vi "EditSine.vi"() -> ()   [LabVIEW 2020, in "Curve Editor.lvlib"]
uses:
  Curve Editor.lvlib
  Key Value/Key Value.lvlib
panel:
  in  "偏移量":dbl format="%.2f"
  in  "相位[度]":dbl format="%.2f"
  in  "幅值":dbl format="%.2f"
  in  "频率":dbl format="%.2f"
  in  "时间[S]":dbl format="%.2f"
  in  "Tree引用句柄":refnum<vi>
  in  "索引":i32
  in  "取消按钮":bool
  in  "确定按钮":bool
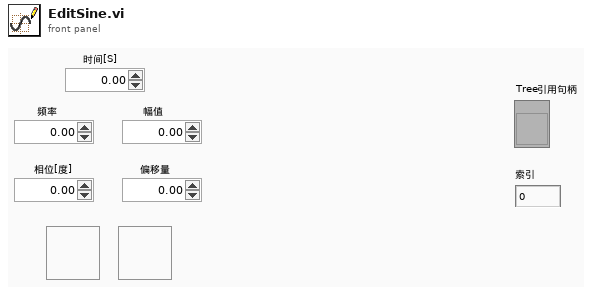
[diagram p1: front panel]
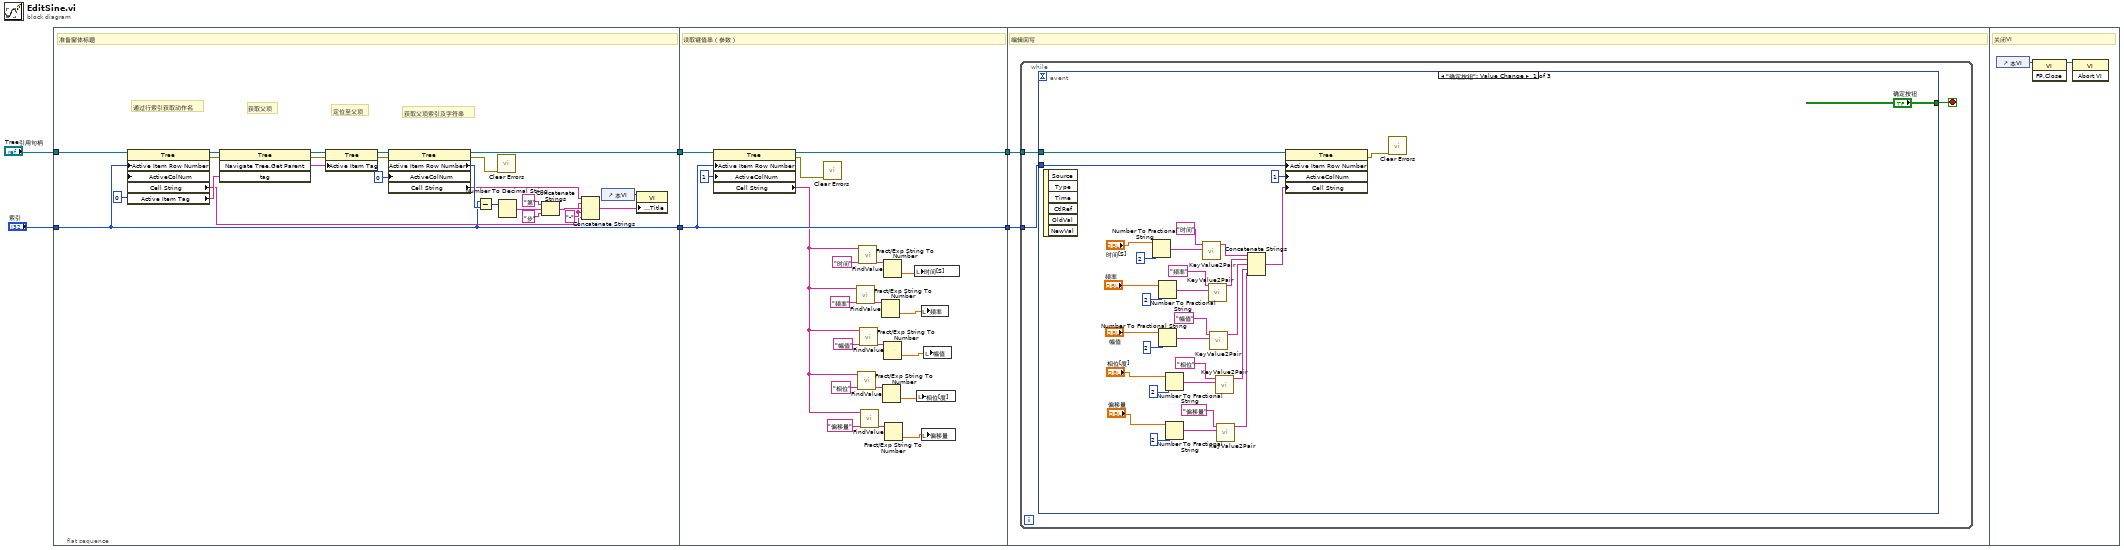
[diagram p0: block diagram]
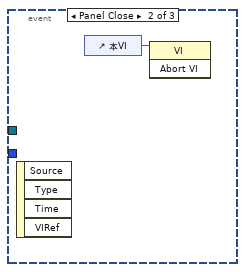
[diagram p2: hidden frame]
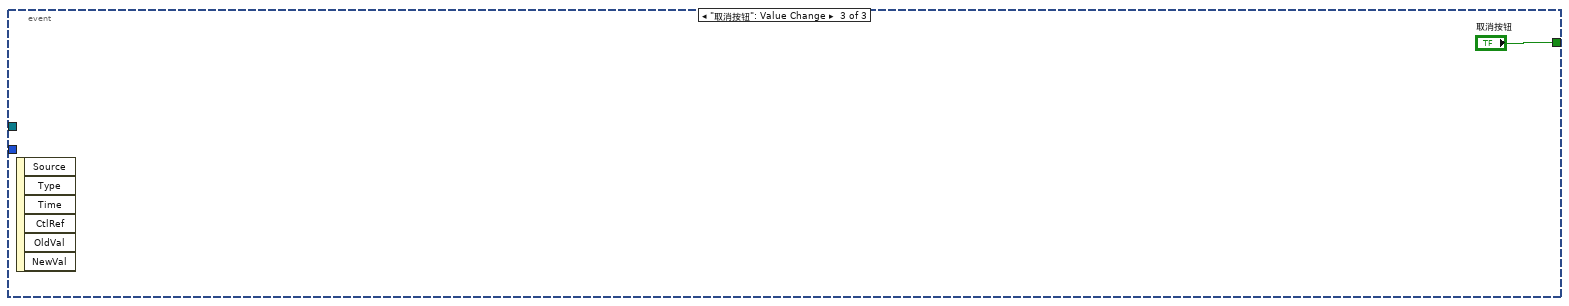
[diagram p3: hidden frame]
diagram:
  n1 = flat-sequence {
    tunnel: [w13] -> w6
    tunnel: [w12] -> w4
    tunnel: "Tree引用句柄" -> [w14]
    tunnel: "索引" -> [w13]
    tunnel: w6 -> [w50]
    tunnel: [w50] -> w5
    tunnel: w4 -> [w51]
    tunnel: [w49] -> w3
    tunnel: w5 -> [w54]
    tunnel: w3 -> [w53]
    frame #0 {
      w16 = "-" ("字符串")
      # "获取父项索引及字符串"
      # "定位至父项"
      # "获取父项"
      # "通过行索引获取动作名"
      # "准备窗体标题"
      n2 = property class="Tree"(reference=w14, "Active Item Row Number"=w13, "ActiveColNum"=0 ("活动单元格:活动列数")) -> (reference out=w11:refnum<vi>, error out=w10:errorcluster, "Cell String"=w15:string, "Active Item Tag"=w28:string)  [unwired: 1 in]
      n3 = invoke class="Tree" method="Navigate Tree.Get Parent"(reference=w11, error in=w10, "tag"=w28) -> (reference out=w23:refnum<vi>, error out=w9:errorcluster, "Navigate Tree:Get Parent"=w24:string)  [unwired: 1 in, 1 out]
      n4 = property class="Tree"(reference=w23, error in=w9, "Active Item Tag"=w24) -> (reference out=w22:refnum<vi>, error out=w8:errorcluster)
      n5 = property class="Tree"(reference=w22, error in=w8, "ActiveColNum"=0 ("活动单元格:活动列数")) -> (reference out=w12:refnum<vi>, error out=w7:errorcluster, "Active Item Row Number"=w26:i32, "Cell String"=w25:string)
      n6 = Subtract(x=w13, y=w26) -> (x-y=w21:i32)
      n7 = call <vilib>:"Clear Errors.vi"("error in (no error)"=w7) -> ()  [unwired: 5 in, 2 out]
      n8 = Number To Decimal String(number=w21) -> (decimal integer string=w19:string)  [unwired: 1 in]
      n9 = Concatenate Strings("第", w19, "步") -> (w17:string)
      n10 = Concatenate Strings(w25, w16, w17, w16, w15) -> (w29:string)
      n11 = control-ref of="本VI"() -> (w31:refnum<vi>)
      n12 = property class="VI"(reference=w31, "Front Panel.Title"=w29) -> ()  [unwired: 1 in, 2 out]
    }
    frame #1 {
      # "读取键值串（参数）"
      n13 = property class="Tree"(reference=w51, "Active Item Row Number"=w50, "ActiveColNum"=1 ("活动单元格:活动列数")) -> (reference out=w49:refnum<vi>, error out=w32:errorcluster, "Cell String"=w33:string)  [unwired: 1 in]
      n14 = call <vilib>:"Clear Errors.vi"("error in (no error)"=w32) -> ()  [unwired: 5 in, 2 out]
      n15 = call "FindValue.vi"("键"="频率", "键值串"=w33) -> ("值"=w44:string)  [unwired: 8 in, 1 out]
      n16 = call "FindValue.vi"("键"="相位", "键值串"=w33) -> ("值"=w38:string)  [unwired: 8 in, 1 out]
      n17 = call "FindValue.vi"("键"="时间", "键值串"=w33) -> ("值"=w47:string)  [unwired: 8 in, 1 out]
      n18 = call "FindValue.vi"("键"="幅值", "键值串"=w33) -> ("值"=w41:string)  [unwired: 8 in, 1 out]
      n19 = call "FindValue.vi"("键"="偏移量", "键值串"=w33) -> ("值"=w35:string)  [unwired: 8 in, 1 out]
      n20 = Fract/Exp String To Number(string=w44) -> (number=w45:dbl)  [unwired: 3 in, 1 out]
      n21 = Fract/Exp String To Number(string=w38) -> (number=w39:dbl)  [unwired: 3 in, 1 out]
      n22 = Fract/Exp String To Number(string=w47) -> (number=w46:dbl)  [unwired: 3 in, 1 out]
      n23 = Fract/Exp String To Number(string=w41) -> (number=w40:dbl)  [unwired: 3 in, 1 out]
      n24 = Fract/Exp String To Number(string=w35) -> (number=w34:dbl)  [unwired: 3 in, 1 out]
      n25 = local write "时间[S]"(w46) -> ()
      n26 = local write "相位[度]"(w39) -> ()
      n27 = local write "频率"(w45) -> ()
      n28 = local write "偏移量"(w34) -> ()
      n29 = local write "幅值"(w40) -> ()
    }
    frame #2 {
      # "编辑回写"
      n30 = while {
        tunnel: w54 -> [w56]
        tunnel: w53 -> [w55]
        stop <- w57 stop-if-true
        n31 = event shown="[0] \"确定按钮\": Value Change" {
          selector: _ -> [_ _ _]
          dyn-events: _ -> [_ _ _]
          timeout: _ -> [_ _ _]
          tunnel: ["确定按钮" _ "取消按钮"] -> w57
          tunnel: w56 -> [w87 _ _]
          tunnel: w55 -> [w86 _ _]
          event "确定按钮": Value Change {
            n32 = event-data() -> ()  [unwired: 1 in, 6 out]
            n33 = Number To Fractional String(number="时间[S]", precision (6)=i16 2 ("精度(6)")) -> (F-format string=w83:string)  [unwired: 2 in]
            n34 = Number To Fractional String(number="频率", precision (6)=i16 2 ("精度(6)")) -> (F-format string=w81:string)  [unwired: 2 in]
            n35 = Number To Fractional String(number="幅值", precision (6)=i16 2 ("精度(6)")) -> (F-format string=w78:string)  [unwired: 2 in]
            n36 = Number To Fractional String(number="相位[度]", precision (6)=i16 2 ("精度(6)")) -> (F-format string=w65:string)  [unwired: 2 in]
            n37 = Number To Fractional String(number="偏移量", precision (6)=i16 2 ("精度(6)")) -> (F-format string=w68:string)  [unwired: 2 in]
            n38 = call "KeyValue2Pair.vi"("值"=w83, "键"="时间") -> ("键值对"=w73:string)  [unwired: 9 in]
            n39 = call "KeyValue2Pair.vi"("值"=w81, "键"="频率") -> ("键值对"=w72:string)  [unwired: 9 in]
            n40 = call "KeyValue2Pair.vi"("值"=w78, "键"="幅值") -> ("键值对"=w71:string)  [unwired: 9 in]
            n41 = call "KeyValue2Pair.vi"("值"=w65, "键"="相位") -> ("键值对"=w61:string)  [unwired: 9 in]
            n42 = call "KeyValue2Pair.vi"("值"=w68, "键"="偏移量") -> ("键值对"=w60:string)  [unwired: 9 in]
            n43 = Concatenate Strings(w73, w72, w71, w61, w60) -> (w70:string)
            n44 = property class="Tree"(reference=w86, "Active Item Row Number"=w87, "ActiveColNum"=1 ("活动单元格:活动列数"), "Cell String"=w70) -> (error out=w58:errorcluster)  [unwired: 1 in, 1 out]
            n45 = call <vilib>:"Clear Errors.vi"("error in (no error)"=w58) -> ()  [unwired: 5 in, 2 out]
          }
          event Panel Close {
            n46 = event-data() -> ()  [unwired: 1 in, 4 out]
            n47 = control-ref of="本VI"() -> (w89:refnum<vi>)
            n48 = invoke class="VI" method="Abort VI"(reference=w89) -> ()  [unwired: 2 in, 3 out]
          }
          event "取消按钮": Value Change {
            n49 = event-data() -> ()  [unwired: 1 in, 6 out]
          }
        }
      }
    }
    frame #3 {
      # "关闭VI"
      n50 = control-ref of="本VI"() -> (w92:refnum<vi>)
      n51 = invoke class="VI" method="FP.Close"(reference=w92) -> (reference out=w91:refnum<vi>)  [unwired: 2 in, 2 out]
      n52 = invoke class="VI" method="Abort VI"(reference=w91) -> ()  [unwired: 2 in, 3 out]
    }
  }
